vi "EEG_2021_099_While Loop.vi"() -> ()   [LabVIEW 2022 SP3]
panel:
  out "Number of iterations":i32
  out "Current Number":dbl
  in  "Number to march":u32=50 max=1000 step=1
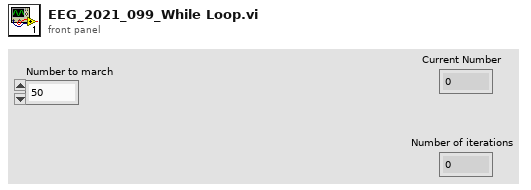
[diagram p1: front panel]
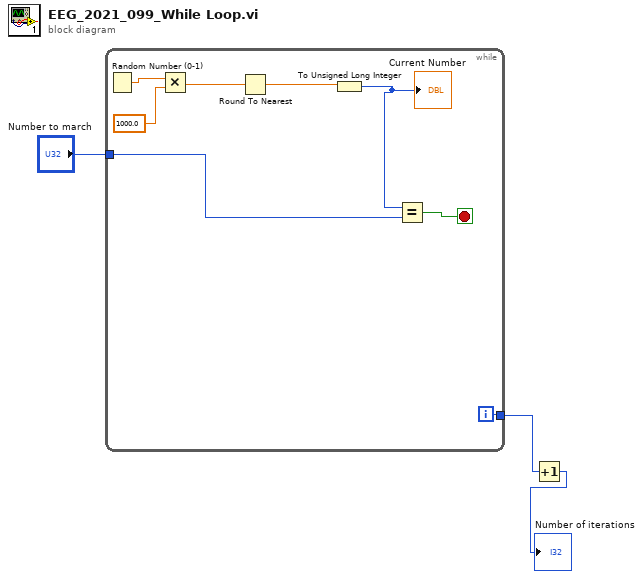
[diagram p0: block diagram]
diagram:
  n1 = while {
    tunnel: "Number to march" -> [w9]
    tunnel: [w6] -> w1
    i -> [w6]
    stop <- w7 stop-if-true
    n2 = Random Number (0-1)() -> (number: 0 to 1=w11:dbl)
    n3 = Multiply(x=w11, y=1000.0 ("x")) -> (x*y=w5:dbl)
    n4 = Round To Nearest(number=w5) -> (nearest integer value=w8:dbl)
    n5 = To Unsigned Long Integer(number=w8) -> (unsigned 32bit integer=w4:u32)
    "Current Number" <- w4
    n6 = Equal?(x=w4, y=w9) -> (x = y?=w7:bool)
  }
  n7 = Increment(x=w1) -> (x+1=→"Number of iterations":i32)
